vi "Test Divide.vi"() -> ()   [LabVIEW 2021]
uses:
  Source/Abs_Types/Double Float/Support/Type.ctl
  Source/Constants/Support/DBL/Const_DBL.lvclass
  C:/TSA/LV_Abstract/Source/Abs_Types/Double Float/Abs_Double Float.lvclass
  C:/Program Files (x86)/National Instruments/LabVIEW 2021/vi.lib/TSA/Abstract Data Classes/Abs_Types/Numeric/Abs_Numeric.lvclass
  Source/Constants/Support/DBL/DBL.vi
  Source/Functions/Math/Support/Divide/DBL/Method.vi
  Source/Abs_Types/Double Float/Abs_Double Float.lvclass
  Source/Functions/Math/Support/Divide/DBL/Divide_DBL.lvclass
  C:/TSA/LV_Abstract/Source/Abs_Types/Floating Point/Abs_Floating Point.lvclass
  C:/Program Files (x86)/National Instruments/LabVIEW 2021/vi.lib/TSA/Abstract Data Classes/Abs_Types/Value/Abs_Value.lvclass
  C:/Program Files (x86)/National Instruments/LabVIEW 2021/vi.lib/TSA/Abstract Data Classes/Abs_Types/Type/Abs_Type.lvclass
  C:/TSA/LV_Abstract/Source/Constants/Support/DBL/Const_DBL.lvclass
panel:
  out "Value":T1
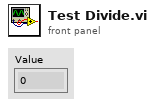
[diagram p1: front panel]
types:
  T1 = typedef "Abs_Double Float.lvclass/Type.ctl" = dbl
  T2 = typedef "Divide_DBL.lvclass/Abs Type.ctl" = refnum<class "Abs_Double Float.lvclass">
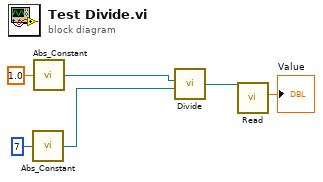
[diagram p0: block diagram]
diagram:
  n1 = call-poly "Abs_Constant.vi"("Value"=7 ("Numeric")) -> ("Constant"=w6:refnum<class "Const_DBL.lvclass">)  [unwired: 4 in]
  n2 = call-poly "Abs_Constant.vi"("Value"=1.0 ("Numeric")) -> ("Constant"=w1:refnum<class "Const_DBL.lvclass">)  [unwired: 4 in]
  n3 = call-poly "Divide.vi"("Input B"=w6, "Input A"=w1) -> ("Result"=w5:T2)  [unwired: 4 in]
  n4 = call-dynamic "Read.vi"("Double Float.lvclass_340760 in"=w5) -> ("Value"=→"Value":T1)  [unwired: 8 in, 2 out]
